vi "IR Polarimeter Software for NIRPol-2.0.vi"() -> ()   [LabVIEW 2017]
uses:
  <vilib>/vision/Image Controls.llb/IMAQ Image.ctl
  <vilib>/Analysis/Matrix/Datatypes/RealMatrix.ctl
  <vilib>/userdefined/High Color/IMAQdx.ctl
  <vilib>/Analysis/baseanly.llb/A x Vector.vi
  <vilib>/Analysis/baseanly.llb/Real A x B.vi
  <vilib>/Instr/_visa.llb/VISA Configure Serial Port (Instr).vi
  <vilib>/Utility/file.llb/Read From Spreadsheet File (DBL).vi
  <vilib>/Utility/file.llb/Write Delimited Spreadsheet (DBL).vi
  <vilib>/gmath/NI_Gmath.lvlib
  <vilib>/Analysis/NI_AALBase.lvlib
  <vilib>/vision/driver/NI_Vision_Acquisition_Software.lvlib
  <vilib>/Analysis/Matrix/NI_Matrix.lvlib
panel:
  out "Abs(cal data - Fit)":dbl[](graph)
  out "Cal Data":dbl[](graph)
  out "Fit":dbl[](graph)
  out "Waveform Chart":dbl(graph)
  out "Numeric":i32
  in  "ROI":i32[](array[numeric])=[155, 255, 103, 203]
  out "IMAQ Session":T1
  out "Camera Handle":T2="cam8"
  in  "Stop Sweeping":bool
  out "Scan Parameters":T3(array[cluster])
  out "cal data and fit":dbl[][][](array[numeric])
  out "Average MM":T4
  out "Dark Img":dbl[][](array[numeric])
  out "Reference Detector Conn":refnum<k21>="RefDetVoltage"
  out "Interface Name":string="img0"
  out "Retarder Motors Driver Output":string
  out "Retarder Motor Driver":refnum<visa-resource-name>
  out "laser VISA Session":refnum<visa-resource-name>
  out "Cal Wavelength":dbl[](array[numeric])
  out "Cal Parameters":dbl[][](array[numeric])
  out "NumWav":dbl=1550.0
  out "Ret Pos":cluster{"Generator":dbl, "Analyzer":dbl}[](array[cluster])
  out "Wavelength List":dbl[](array[numeric])
  out "inverse MM":dbl[][][](array[numeric])
  out "Dark Ref":dbl format="%0.2f"
  out "Reference Detector Reading":string
  out "Reference Detector Value":dbl format="%0.9f"
  out "Image Out":T1
  out "Image Pixels (I16)":i16[][](array[numeric])
  out "Mean":dbl
  out "Minimum":i16
  out "Maximum":i16
  out "Camera Output":i16[][](graph)
  in  "Tab Control":T5(tab)
  in  "Calibrate":bool
  in  "Save calibration file:":path=path "C:/Users/DTS20/Desktop/NIRPOL Revision"
  in  "Load calibration file:":path=path "C:/Users/DTS20/Desktop/NIRPOL Revision/caldata"
  in  "Set Wavelengths:":dbl[][](array[numeric])=[[1550.0]]
  in  "Use User-Defined Retarder Positions?":bool
  in  "Load User-Defined Retarder Positions (optional):":path
  in  "Start Measurement":bool
  in  "Save Mueller Matrix Output To (folder):":path=path "J:/Users/Lisa/foo"
  in  "Use MM Inverse?":bool
  in  "Comments":string
  in  "Use Reference Detector:":bool
  in  "Images to Average":i32=10
  in  "+/-":dbl
  in  "Sweep wavelength?":bool
  in  "Laser On/Off":bool
  in  "Update Camera":bool
  in  "Laser Power [mW]":dbl=6.0 format="%.2f"
  in  "Wavelength [nm]":dbl=1550.0
  in  "Update Laser Source":bool
  in  "PSG Retarder Angle":dbl
  in  "PSA Retarder Angle":dbl
  in  "Update Retarder Angles":bool
  in  "Home Ret Motors":bool
  in  "Exposure [µs]":dbl=1000.0
  in  "Binning":i32=1
  # "Min X"
  # "Max X"
  # "Min Y"
  # "Max Y"
  # "Sweep Wavelength\nDuring Measurement"
  # "AOI"
  # "AOS"
  # "nm"
  # "General Options:"
  # "Laser Control:"
  # "Retarder Motor Control:"
  # "Camera Control"
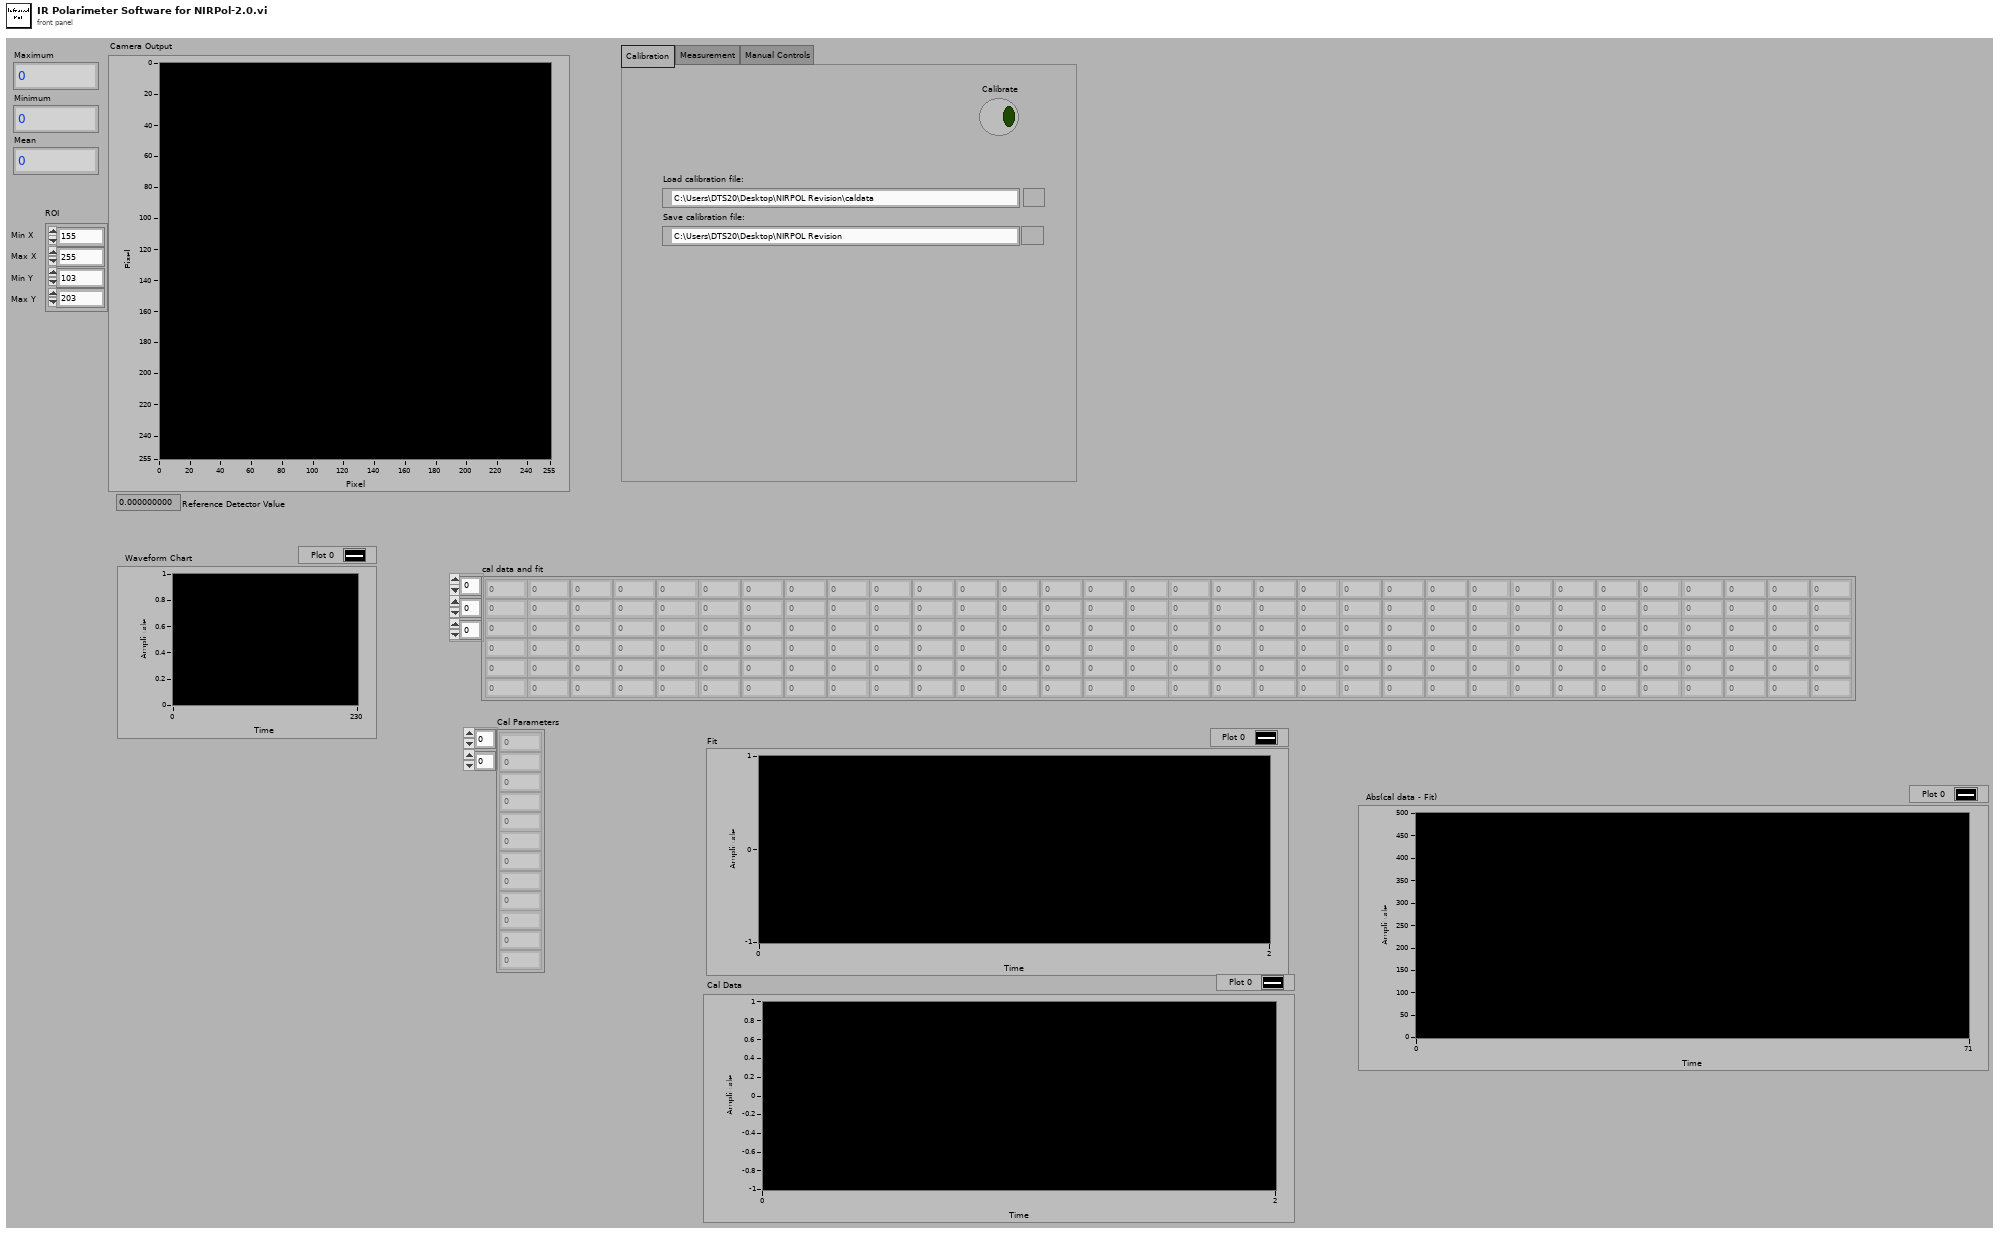
[diagram p1: front panel]
types:
  T1 = typedef "IMAQ Image.ctl" = refnum<image>
  T2 = typedef "IMAQdx.ctl" = refnum<k21>
  T3 = cluster{"Wavelength":dbl, "PSG Angle":dbl, "PSA Angle":dbl}[]
  T4 = typedef "NI_Matrix.lvlib/RealMatrix.ctl" = dbl[][]
  T5 = enum32{"Calibration", "Measurement", "Manual Controls"}
  T6 = enum16{"big-endian, network order", "native, host order", "little-endian"}
  T7 = cluster{"wavelength":dbl, "amplitude":dbl, "gen leakage":dbl, "an leakage":dbl, "generator retardance":dbl, "analyzer retardance":dbl, "gen offset":dbl, "an offset":dbl, "an pol offset":dbl}[]
  T8 = cluster{"Wavelength":dbl, "Camera Arm":dbl, "Source Arm":dbl}[]
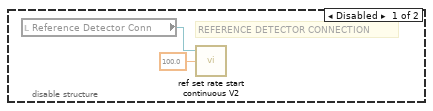
[diagram p2: hidden frame]
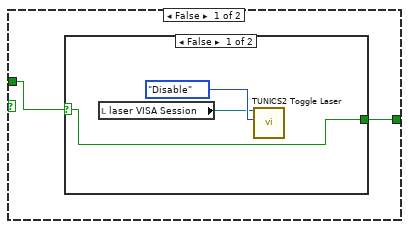
[diagram p3: hidden frame]
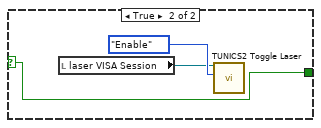
[diagram p4: hidden frame]
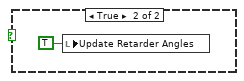
[diagram p5: hidden frame]
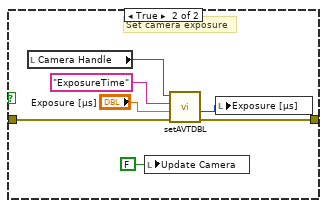
[diagram p6: hidden frame]
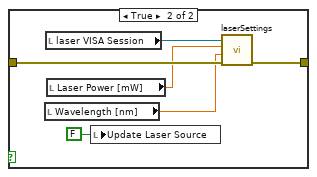
[diagram p7: hidden frame]
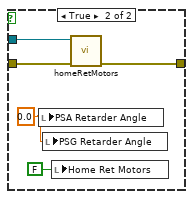
[diagram p9: hidden frame]
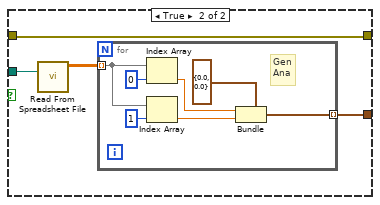
[diagram p10: hidden frame]
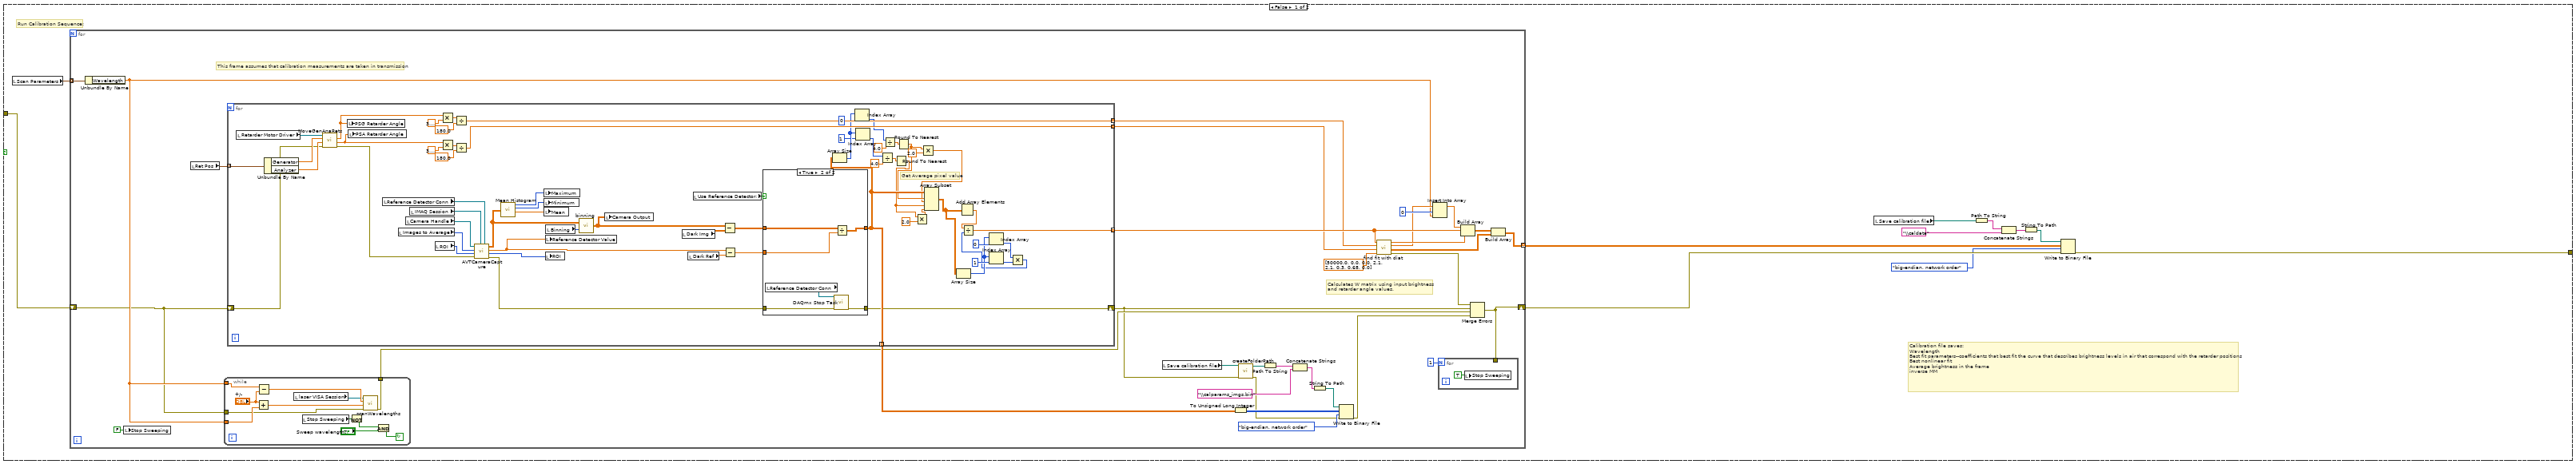
[diagram p11: hidden frame]
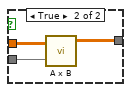
[diagram p13: hidden frame]
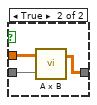
[diagram p14: hidden frame]
diagram:
  # "In This Frame:\n1.) Play a pleasant \"finished\" tone.\n2.) Home retarder motors\n3.) Home arm motors"
  # "In This Frame: Setup for measurement or calibration\n1.) Disable laser to take a dark measurement\n2.) Clear all IMAQ images\n3.) Capture a dark image (to be subtracted from each frame)\n4.) Construct a List of wavelengths and AOI-AOS from user input\n5.) Enable the laser again after a dark measurement\n6.) Load user-defined retarder positions and construct a cluster"
  # "Hidden Constants:"
  # "Display Indicators:"
  # "Numerical Controls:"
  # "Buttons:"
  # "Connections:"
  # "In This Frame:\n1) Initialize the laser\n2) Initialize and home retarder motors\n3) Initialize camera connection\nTODO: Init connection w/ ref detector"
  # "In This Frame:\nContinous Updates are done while the system is setup and prepared for measurement.\n1) Create a bad pixel map\n2) Manually set or home retarder motors\n3) Manually set or home arm motor positions\n4) Manually control laser brightness or wavelength\n5) Continusly Capture camera frames."
  n1 = flat-sequence {
    tunnel: [w38] -> w6
    tunnel: w6 -> [w61]
    tunnel: [w63] -> w2
    tunnel: [w156] -> w5
    tunnel: w2 -> [w146]
    tunnel: w5 -> [w212]
    tunnel: [w211] -> w4
    tunnel: w4 -> [w600]
    frame #0 {
      w16 = 180
      w17 = 3.1416
      w33 = errorcluster {"status"=FALSE, "code"=0, "source"=""} ("error in (no error)")
      w44 = u16 0 items=["None", "XON/XOFF", "RTS/CTS", "XON/XOFF & RTS/CTS", "DTR/DSR", "XON/XOFF & DTR/DSR"] ("flow control (0:none)")
      w47 = u16 10 items=["1.0"=10, "1.5"=15, "2.0"=20] ("stop bits (10: 1 bit)")
      # "RETARDER MOTOR INITIALIZATION"
      # "ILLUMINATION SOURCE CONNECTION"
      # "RETARDER MOTOR CONNECTION"
      # "In This Frame:\nInitialize contact with all hardware needed in system"
      n2 = local read "Camera Handle"() -> (w31:T2)
      n3 = local read "laser VISA Session"() -> (w42:refnum<visa-resource-name>)
      n4 = local read "Retarder Motor Driver"() -> (w43:refnum<visa-resource-name>)
      n5 = call "IMAQ Create"("Image Name"="Grab", "error in (no error)"=w33) -> ("New Image"=→"IMAQ Session":T1, "error out"=w32:errorcluster)  [unwired: 3 in]
      n6 = call <vilib>:"IMAQdx Open Camera.vi"("error in"=w33, "Session In"=w31) -> ("error out"=w36:errorcluster, "Session Out"=w35:T2)  [unwired: 8 in]
      n7 = call "TUNICS2 Toggle Laser.vi"("error in (no error)"=w33, "Laser Output (Disable:0)"=enum16{"Enable", "Disable"}."Enable", "VISA resource name"=w42) -> ("error out"=w39:errorcluster)  [unwired: 3 in, 1 out]
      n8 = call <vilib>:"IMAQdx Configure Grab.vi"("error in"=w36, "Session In"=w35) -> ("error out"=w34:errorcluster)  [unwired: 8 in, 1 out]
      n9 = disable-structure shown="Enabled" {
        frame Disabled {
          # "REFERENCE DETECTOR CONNECTION"
          n10 = local read "Reference Detector Conn"() -> (w57:refnum<k21>)
          n11 = call "ref set rate start continuous V2.vi"("rate (S/s)"=100.0, "task/channels in"=w57) -> ()  [unwired: 1 in, 2 out]
        }
        frame Enabled {
        }
      }
      n12 = local read "Load calibration file:"() -> (w29:path)
      n13 = call-poly "VISA Configure Serial Port"("VISA resource name"=w43, "timeout (10sec)"=u32 1, "termination char\n(0xA = '\\n' = LF)"=u8 10 ("termination char\n(0xA = '\\n' = LF)"), "Enable Termination\nChar (T)"=TRUE ("Enable Termination\nChar (T)"), "baud rate (9600)"=u32 9600, "data bits (8)"=u16 8, "parity (0:none)"=enum16{"None", "Odd", "Even", "Mark", "Space"}."Even", "error in (no error)"=w33, "stop bits (10: 1 bit)"=w47, "flow control (0:none)"=w44) -> ("error out"=w25:errorcluster)  [unwired: 4 in, 1 out]
      n14 = call "LoadCalwDiat.vi"("file (use dialog)"=w29, "error in"=w25) -> ("Calibration params"=w26:T7, "error out"=w28:errorcluster)  [unwired: 2 out]
      n15 = flat-sequence {
        tunnel: w24 -> [w60]
        tunnel: [w58] -> w40
        tunnel: w10 -> [_]
        tunnel: w12 -> [_]
        frame #0 {
          # "01: Gen\n02: Ana"
          # "Homing retarder motors\nSetting arm motors  limits and homing"
          n16 = local read "Retarder Motor Driver"() -> (w59:refnum<visa-resource-name>)
          n17 = call "homeRetMotors.vi"("error in (no error)"=w60, "VISA Refnum in"=w59) -> ("error out"=w58:errorcluster)  [unwired: 9 in]
        }
      }
      n18 = for {
        N: 1 -> [_]
        shift-right: [w52] -> w24
        shift-left: w28 -> [w52]
        tunnel: [w54] -> w23 mode=indexing
        tunnel: [w53] -> w22 mode=indexing
        tunnel: w26 -> [w55] mode=indexing
        n19 = Unbundle By Name(w55) -> ("gen offset"=w54:dbl, "an offset"=w53:dbl)
        n20 = call <vilib>:"Simple Error Handler.vi"("error in (no error)"=w52) -> ()  [unwired: 4 in, 5 out]
      }
      n21 = Negate(x=w23) -> (-x=w21:dbl[])
      n22 = Negate(x=w22) -> (-x=w18:dbl[])
      n23 = Index Array(array=w21, index=0) -> (element=w15:dbl)
      n24 = Index Array(array=w18, index=0) -> (element=w14:dbl)
      n25 = Divide(x=w15, y=w17) -> (x/y=w11:dbl)
      n26 = Divide(x=w14, y=w17) -> (x/y=w13:dbl)
      n27 = Multiply(x=w13, y=w16) -> (x*y=w12:dbl)
      n28 = Multiply(x=w11, y=w16) -> (x*y=w10:dbl)
      n29 = Merge Errors(w39, w33, w40, w34, w32) -> (w38:errorcluster)
      n30 = call <vilib>:"Simple Error Handler.vi"("error in (no error)"=w38) -> ()  [unwired: 4 in, 5 out]
    }
    frame #1 {
      n31 = while {
        shift-right: [w64] -> w63
        shift-left: w61 -> [w87]
        shift-right: [w68] -> _
        shift-left: TRUE ("Laser On/Off") -> [w70]
        i -> [w74]
        stop <- w90 stop-if-true
        # "Camera Capture and Reference Detector Value"
        # "In This Frame:\nUpdate laser power and brightness"
        # "In This Frame:\nUpdate retarder motor angles if maually changed"
        # "In This Frame:\nHome retarder motors"
        n32 = local read "Laser On/Off"() -> (w69:bool)
        n33 = Equal?(x=0, y=w74) -> (x = y?=w72:bool)
        n34 = Equal?(x=w69, y=w70) -> (x = y?=w71:bool)
        n35 = case shown="False" w72 {
          frame False {
          }
          frame True {
            n36 = local write "Update Retarder Angles"(TRUE ("Update Retarder Angles")) -> ()
          }
        }
        n37 = case shown="True" w71 {
          tunnel: w69 -> [w100 w107]
          tunnel: [w99 w107] -> w68
          frame False {
            n38 = case shown="False" w100 {
              selector: w100 -> [w101 w104]
              tunnel: [w101 w104] -> w99
              frame False {
                n39 = local read "laser VISA Session"() -> (w102:refnum<visa-resource-name>)
                n40 = call "TUNICS2 Toggle Laser.vi"("Laser Output (Disable:0)"=enum16{"Enable", "Disable"}."Disable", "VISA resource name"=w102) -> ()  [unwired: 4 in, 2 out]
              }
              frame True {
                n41 = local read "laser VISA Session"() -> (w105:refnum<visa-resource-name>)
                n42 = call "TUNICS2 Toggle Laser.vi"("Laser Output (Disable:0)"=enum16{"Enable", "Disable"}."Enable", "VISA resource name"=w105) -> ()  [unwired: 4 in, 2 out]
              }
            }
          }
          frame True {
          }
        }
        n43 = case shown="False" "Update Camera" {
          tunnel: w87 -> [w109 w116]
          tunnel: [w109 w115] -> w82
          frame False {
          }
          frame True {
            # "Set camera exposure"
            n44 = local read "Camera Handle"() -> (w110:T2)
            n45 = local write "Update Camera"(FALSE ("Update Camera")) -> ()
            n46 = call "setAVTDBL.vi"("error in (no error)"=w116, "Value In"="Exposure [µs]", "ActiveAttribute"="ExposureTime", "Camera Session In"=w110) -> ("error out"=w115:errorcluster, "Value Out"=w112:u32)  [unwired: 5 in, 1 out]
            n47 = local write "Exposure [µs]"(w112) -> ()
          }
        }
        n48 = local read "Retarder Motor Driver"() -> (w93:refnum<visa-resource-name>)
        n49 = local read "Home Ret Motors"() -> (w96:bool)
        n50 = local read "Reference Detector Conn"() -> (w75:refnum<k21>)
        n51 = case shown="False" w96 {
          tunnel: w87 -> [w133 w137]
          tunnel: [w133 w136] -> w94
          tunnel: w93 -> [_ w138]
          frame False {
          }
          frame True {
            w135 = 0.0 ("Analyzer Angle")
            n52 = local write "PSA Retarder Angle"(w135) -> ()
            n53 = local write "PSG Retarder Angle"(w135) -> ()
            n54 = local write "Home Ret Motors"(FALSE ("Home Ret Motors")) -> ()
            n55 = call "homeRetMotors.vi"("error in (no error)"=w137, "VISA Refnum in"=w138) -> ("error out"=w136:errorcluster)  [unwired: 9 in]
          }
        }
        n56 = local read "Images to Average"() -> (w78:i32)
        n57 = local read "Camera Handle"() -> (w77:T2)
        n58 = local read "IMAQ Session"() -> (w76:T1)
        n59 = local read "Binning"() -> (w89:i32)
        n60 = call "AVTCameraCapture.vi"("Reference Detector Conn"=w75, "IMAQ Session"=w76, "error in (no error)"=w82, "ROI In"="ROI", "Images to Average"=w78, "Camera Handle"=w77) -> ("error out"=w65:errorcluster, "ROI Out"=w80:i32[], "Reference Detector Value"=w67:dbl, "Camera Output"=w79:dbl[][])
        "Waveform Chart" <- w67
        n61 = local write "Reference Detector Value"(w67) -> ()
        n62 = local write "ROI"(w80) -> ()
        n63 = call "binning.vi"("Binning"=w89, "Unbinned"=w79) -> ("Binned array"=w88:dbl[][])
        n64 = call "Mean Histogram.vi"("Array"=w79) -> ("max value"=w83:i16, "min value"=w85:i16, "mean val"=w84:dbl)  [unwired: 3 out]
        n65 = case shown="True" "Update Retarder Angles" {
          tunnel: w93 -> [_ w131]
          tunnel: [w124 w130] -> w92
          tunnel: w94 -> [w124 w132]
          frame False {
          }
          frame True {
            n66 = local read "PSG Retarder Angle"() -> (w128:dbl)
            n67 = local read "PSA Retarder Angle"() -> (w127:dbl)
            n68 = local write "Update Retarder Angles"(FALSE ("Update Retarder Angles")) -> ()
            n69 = call "MoveGenAnaRets.vi"("error in (no error)"=w132, "Analyzer In"=w127, "Generator In"=w128, "VISA resource name"=w131) -> ("error out"=w130:errorcluster, "Analyzer Out"=w126:dbl, "Generator Out"=w125:dbl)  [unwired: 1 out]
            n70 = local write "PSA Retarder Angle"(w126) -> ()
            n71 = local write "PSG Retarder Angle"(w125) -> ()
          }
        }
        n72 = local write "Minimum"(w85) -> ()
        n73 = local write "Mean"(w84) -> ()
        n74 = local write "Camera Output"(w88) -> ()
        n75 = local write "Maximum"(w83) -> ()
        n76 = local read "Update Laser Source"() -> (w91:bool)
        n77 = case shown="False" w91 {
          tunnel: w92 -> [w117 w123]
          tunnel: [w117 w122] -> w66
          frame False {
          }
          frame True {
            n78 = local read "Wavelength [nm]"() -> (w120:dbl)
            n79 = local read "laser VISA Session"() -> (w119:refnum<visa-resource-name>)
            n80 = local read "Laser Power [mW]"() -> (w121:dbl)
            n81 = local write "Update Laser Source"(FALSE ("Update Laser Source")) -> ()
            n82 = call "laserSettings.vi"("error in (no error)"=w123, "Wavelength [nm]"=w120, "Laser Power [mW]"=w121, "VISA Refnum in"=w119) -> ("error out"=w122:errorcluster)  [unwired: 1 in, 2 out]
          }
        }
        n83 = local read "Start Measurement"() -> (w98:bool)
        n84 = local read "Calibrate"() -> (w97:bool)
        n85 = Or(x=w98, y=w97) -> (x .or. y?=w90:bool)
        n86 = Merge Errors(w66, w65) -> (w64:errorcluster)
        n87 = call <vilib>:"Simple Error Handler.vi"("error in (no error)"=w64) -> ()  [unwired: 4 in, 5 out]
      }
    }
    frame #2 {
      w144 = 0.0 ("Generator In")
      # "Set scanning parameters:\nThis subVI creates an array of clusters which contain the wavelength and\nscatter angles for each Mueller matrix in the scan"
      # "Capture dark image"
      # "Enable Laser again after the\ndark measurement"
      # "Disable laser to take dark measurement"
      # "If the user desires, they can load an pre-defined retarder angles from an excel doc or csv. Otherwise, a default set of 64 positions is constructed where the PSA rotates 4.9x as fast as the PSG"
      n88 = local read "Retarder Motor Driver"() -> (w143:refnum<visa-resource-name>)
      n89 = call "MoveGenAnaRets.vi"("error in (no error)"=w146, "Analyzer In"=w144, "Generator In"=w144, "VISA resource name"=w143) -> ("error out"=w145:errorcluster, "Analyzer Out"=w148:dbl, "Generator Out"=w147:dbl)  [unwired: 1 out]
      n90 = local write "PSA Retarder Angle"(w148) -> ()
      n91 = local write "PSG Retarder Angle"(w147) -> ()
      n92 = local read "laser VISA Session"() -> (w154:refnum<visa-resource-name>)
      n93 = call "TUNICS2 Toggle Laser.vi"("error in (no error)"=w145, "Laser Output (Disable:0)"=enum16{"Enable", "Disable"}."Disable", "VISA resource name"=w154) -> ("error out"=w151:errorcluster)  [unwired: 3 in, 1 out]
      n94 = flat-sequence {
        tunnel: w151 -> [w167]
        tunnel: [w167] -> w149
        tunnel: w149 -> [w180]
        tunnel: [w179] -> w142
        tunnel: [w185] -> w150
        tunnel: w142 -> [w185]
        frame #0 {
          n95 = Wait (ms)(milliseconds to wait=u32 1000) -> ()  [unwired: 1 out]
        }
        frame #1 {
          # "Save as dark image"
          n96 = local read "Reference Detector Conn"() -> (w174:refnum<k21>)
          n97 = local read "Images to Average"() -> (w177:i32)
          n98 = local read "Camera Handle"() -> (w176:T2)
          n99 = local read "IMAQ Session"() -> (w175:T1)
          n100 = local read "ROI"() -> (w178:i32[])
          n101 = call "AVTCameraCapture.vi"("Reference Detector Conn"=w174, "IMAQ Session"=w175, "error in (no error)"=w180, "ROI In"=w178, "Images to Average"=w177, "Camera Handle"=w176) -> ("error out"=w179:errorcluster, "ROI Out"=w173:i32[], "Reference Detector Value"=w168:dbl, "Camera Output"=w172:dbl[][])
          n102 = local read "Binning"() -> (w181:i32)
          n103 = local write "Dark Ref"(w168) -> ()
          n104 = local write "ROI"(w173) -> ()
          n105 = call "Mean Histogram.vi"("Array"=w172) -> ("max value"=w171:i16, "min value"=w170:i16, "mean val"=w169:dbl)  [unwired: 3 out]
          n106 = local write "Waveform Chart"(w168) -> ()
          n107 = local write "Minimum"(w170) -> ()
          n108 = local write "Maximum"(w171) -> ()
          n109 = local write "Mean"(w169) -> ()
          n110 = call "binning.vi"("Binning"=w181, "Unbinned"=w172) -> ("Binned array"=w182:dbl[][])
          n111 = local write "Camera Output"(w182) -> ()
          n112 = local write "Dark Img"(w182) -> ()
        }
        frame #2 {
          n113 = for {
            N: 10 -> [_]
            tunnel: [w186] -> w183
            i -> [w186]
            n114 = Wait (ms)(milliseconds to wait=u32 1000) -> ()  [unwired: 1 out]
          }
          "Numeric" <- w183
        }
      }
      n115 = call "setScanParams.vi"("error in (no error)"=w150, "Set Wavelengths:"="Set Wavelengths:") -> ("error out"=w141:errorcluster, "Scan Parameters"=→"Scan Parameters":T8)  [unwired: 8 in]
      n116 = flat-sequence {
        tunnel: w141 -> [w163]
        tunnel: [w162] -> w139
        tunnel: [w165] -> w140
        tunnel: w139 -> [w165]
        frame #0 {
          n117 = local read "laser VISA Session"() -> (w160:refnum<visa-resource-name>)
          n118 = call "TUNICS2 Toggle Laser.vi"("error in (no error)"=w163, "Laser Output (Disable:0)"=enum16{"Enable", "Disable"}."Enable", "VISA resource name"=w160) -> ("error out"=w162:errorcluster)  [unwired: 3 in, 1 out]
        }
        frame #1 {
          n119 = Wait (ms)(milliseconds to wait=u32 60000) -> ()  [unwired: 1 out]
        }
      }
      n120 = case shown="False" "Use User-Defined Retarder Positions?" {
        tunnel: [w189 w201] -> w158
        tunnel: "Load User-Defined Retarder Positions (optional):" -> [_ w203]
        tunnel: w140 -> [w188 w200]
        tunnel: [w188 w200] -> w156
        frame False {
          n121 = for {
            N: 64 -> [w198]
            tunnel: [w191] -> w189 mode=indexing
            i -> [w196]
            n122 = Divide(x=360.0, y=w198) -> (x/y=w197:dbl)
            n123 = Multiply(x=w197, y=w196) -> (x*y=w194:dbl)
            n124 = Multiply(x=w194, y=4.9) -> (x*y=w193:dbl)
            n125 = Bundle(cluster=cluster{"x":dbl, "x 2":dbl} {"x"=0.0, "x 2"=0.0} ("input cluster"), "x"=w193, "x 2"=w194) -> (w191:cluster{"x":dbl, "x 2":dbl})
          }
        }
        frame True {
          n126 = call-poly <vilib>:"Read From Spreadsheet File.vi"("file path (dialog if empty)"=w203) -> ("all rows"=w202:dbl[][])  [unwired: 6 in, 4 out]
          n127 = for {
            tunnel: w202 -> [w208] mode=indexing
            tunnel: [w204] -> w201 mode=indexing
            # "Gen\nAna"
            n128 = Index Array(array=w208, index=0) -> (element=w206:dbl)
            n129 = Index Array(array=w208, index=1) -> (element=w205:dbl)
            n130 = Bundle(cluster=cluster{"x":dbl, "x 2":dbl} {"x"=0.0, "x 2"=0.0} ("input cluster"), "x"=w206, "x 2"=w205) -> (w204:cluster{"x":dbl, "x 2":dbl})
          }
        }
      }
      n131 = local write "Ret Pos"(w158) -> ()
    }
    frame #3 {
      # "In This Frame: Run a measurement or a calibration"
      n132 = local read "Start Measurement"() -> (w213:bool)
      n133 = case shown="True" w213 {
        tunnel: w212 -> [w224 w365]
        tunnel: [w220 w359] -> w211
        frame False {
          # "Calibration file saves:\nWavelength\nBest fit parameters--coefficients that best fit the curve that describes brightness levels in air that correspond with the retarder positions\nBest nonlinear fit\nAverage brightness in the frame\ninverse MM"
          # "Run Calibration Sequence:"
          n134 = local read "Scan Parameters"() -> (w219:T3)
          n135 = for {
            tunnel: [w249] -> w221 mode=indexing
            shift-right: [w240] -> w223
            shift-left: w224 -> [w227]
            tunnel: w219 -> [w244] mode=indexing
            # "Calculates W matrix using input brightness\nand retarder angle values."
            # "This frame assumes that calibration measurements are taken in transmission"
            n136 = Unbundle By Name(w244) -> ("Wavelength"=w242:dbl)
            n137 = local write "Stop Sweeping"(FALSE ("stop scanning")) -> ()
            n138 = local read "Ret Pos"() -> (w254:cluster{"Generator":dbl, "Analyzer":dbl}[])
            n139 = while {
              tunnel: w242 -> [w269]
              tunnel: w242 -> [w267]
              tunnel: w227 -> [w259]
              tunnel: [w258] -> w226
              stop <- w261 continue-if-true
              n140 = Add(x="+/-", y=w269) -> (x+y=w268:dbl)
              n141 = Subtract(x=w267, y="+/-") -> (x-y=w265:dbl)
              n142 = local read "laser VISA Session"() -> (w260:refnum<visa-resource-name>)
              n143 = local read "Stop Sweeping"() -> (w264:bool)
              n144 = Not(x=w264) -> (.not. x?=w263:bool)
              n145 = call "scanWavelengths.vi"("error in (no error)"=w259, "Start Wavelength [nm]"=w268, "End Wavelength [nm]"=w265, "VISA Refnum in"=w260) -> ("error out"=w258:errorcluster)  [unwired: 7 in]
              n146 = And(x=w263, y="Sweep wavelength?") -> (x .and. y?=w261:bool)
            }
            n147 = for {
              tunnel: [w330] -> w252 mode=indexing
              shift-right: [w271] -> w225
              shift-left: w227 -> [w302]
              tunnel: w254 -> [w318] mode=indexing
              tunnel: [w312] -> w245 mode=indexing
              tunnel: [w308] -> w246 mode=indexing
              tunnel: [w284] -> w238 mode=indexing
              # "Get Average pixel value"
              n148 = local read "Retarder Motor Driver"() -> (w305:refnum<visa-resource-name>)
              n149 = Unbundle By Name(w318) -> ("Generator"=w304:dbl, "Analyzer"=w303:dbl)
              n150 = call "MoveGenAnaRets.vi"("error in (no error)"=w302, "Analyzer In"=w303, "Generator In"=w304, "VISA resource name"=w305) -> ("error out"=w291:errorcluster, "Analyzer Out"=w300:dbl, "Generator Out"=w301:dbl)  [unwired: 1 out]
              n151 = local write "PSG Retarder Angle"(w301) -> ()
              n152 = local write "PSA Retarder Angle"(w300) -> ()
              n153 = local read "Reference Detector Conn"() -> (w270:refnum<k21>)
              n154 = local read "Images to Average"() -> (w293:i32)
              n155 = local read "Camera Handle"() -> (w294:T2)
              n156 = local read "IMAQ Session"() -> (w295:T1)
              n157 = local read "ROI"() -> (w292:i32[])
              n158 = Multiply(x=w301, y=3.141592653589793) -> (x*y=w314:dbl)
              n159 = Multiply(x=w300, y=3.141592653589793) -> (x*y=w310:dbl)
              n160 = Divide(x=w314, y=180.0) -> (x/y=w312:dbl)
              n161 = Divide(x=w310, y=180.0) -> (x/y=w308:dbl)
              n162 = call "AVTCameraCapture.vi"("Reference Detector Conn"=w270, "IMAQ Session"=w295, "error in (no error)"=w291, "ROI In"=w292, "Images to Average"=w293, "Camera Handle"=w294) -> ("error out"=w289:errorcluster, "ROI Out"=w297:i32[], "Reference Detector Value"=w290:dbl, "Camera Output"=w299:dbl[][])
              n163 = call "Mean Histogram.vi"("Array"=w299) -> ("max value"=w316:i16, "min value"=w317:i16, "mean val"=w296:dbl)  [unwired: 3 out]
              n164 = local write "Maximum"(w316) -> ()
              n165 = local write "Minimum"(w317) -> ()
              n166 = local write "Mean"(w296) -> ()
              n167 = local write "Reference Detector Value"(w290) -> ()
              n168 = local write "ROI"(w297) -> ()
              n169 = local read "Binning"() -> (w306:i32)
              n170 = call "binning.vi"("Binning"=w306, "Unbinned"=w299) -> ("Binned array"=w298:dbl[][])
              n171 = local write "Camera Output"(w298) -> ()
              n172 = local read "Dark Img"() -> (w307:dbl[][])
              n173 = local read "Dark Ref"() -> (w322:dbl)
              n174 = local read "Use Reference Detector:"() -> (w319:bool)
              n175 = Subtract(x=w298, y=w307) -> (x-y=w323:dbl[][])
              n176 = Subtract(x=w290, y=w322) -> (x-y=w321:dbl)
              n177 = case shown="True" w319 {
                tunnel: w323 -> [w332 w338]
                tunnel: w321 -> [_ w337]
                tunnel: [w332 w336] -> w284
                tunnel: w289 -> [w331 w335]
                tunnel: [w331 w333] -> w271
                frame False {
                }
                frame True {
                  n178 = local read "Reference Detector Conn"() -> (w334:refnum<k21>)
                  n179 = call <vilib>:"DAQmx Stop Task.vi"("task/channels in"=w334, "error in"=w335) -> ("error out"=w333:errorcluster)  [unwired: 12 in, 1 out]
                  n180 = Divide(x=w338, y=w337) -> (x/y=w336:dbl[][])
                }
              }
              n181 = Array Size(array=w284) -> (size(s)=w288:i32[])
              n182 = Index Array(array=w288, index=0) -> (element=w282:i32)
              n183 = Index Array(array=w288, index=1) -> (element=w280:i32)
              n184 = Divide(x=w280, y=4.0) -> (x/y=w279:dbl)
              n185 = Divide(x=w282, y=4.0) -> (x/y=w278:dbl)
              n186 = Round To Nearest(number=w279) -> (nearest integer value=w273:dbl)
              n187 = Round To Nearest(number=w278) -> (nearest integer value=w277:dbl)
              n188 = Multiply(x=w273, y=2.0) -> (x*y=w272:dbl)
              n189 = Multiply(x=w277, y=2.0) -> (x*y=w275:dbl)
              n190 = Array Subset "Array Subset"(array=w284, index (row)=w277, length (row)=w275, index (col)=w273, length (col)=w272) -> (w285:dbl[][])
              n191 = Array Size(array=w285) -> (size(s)=w327:i32[])
              n192 = Add Array Elements(numeric array=w285) -> (sum=w320:dbl)
              n193 = Index Array(array=w327, index=0) -> (element=w325:i32)
              n194 = Index Array(array=w327, index=1) -> (element=w326:i32)
              n195 = Multiply(x=w325, y=w326) -> (x*y=w324:i32)
              n196 = Divide(x=w320, y=w324) -> (x/y=w330:dbl)
            }
            n197 = local read "Save calibration file:"() -> (w236:path)
            n198 = To Unsigned Long Integer(number=w238) -> (unsigned 32bit integer=w237:u32[][][])
            n199 = call "createFolderPath.vi"("error in (no error)"=w225, "File Path Control"=w236) -> ("error out"=w229:errorcluster, "Path"=w235:path)  [unwired: 8 in]
            n200 = Path To String(path=w235) -> (string=w234:string)
            n201 = Concatenate Strings(w234, "\\calparams_imgs.bin") -> (w232:string)
            n202 = String To Path(string=w232) -> (path=w231:path)
            n203 = Write to Binary File(file (use dialog)=w231, data=w237, error in=w229, 9:T6."big-endian, network order" ("byte order (0:big-endian, network order)")) -> (error out=w228:errorcluster)  [unwired: 2 in, 2 out]
            n204 = call "find fit with diat.vi"("initial parameters"=dbl[] [50000.0, 0.0, 0.0, 2.1, 2.1, 0.3, 0.68, 0.0], "t2"=w246, "t1"=w245, "Y"=w252) -> ("error out"=w239:errorcluster, "inverse MM"=w248:dbl[][], "best fit parameters"=w250:dbl[], "best nonlinear fit"=w251:dbl[])
            n205 = Insert Into Array(array=w250, index=0, new element=w242) -> (w256:dbl[])
            n206 = Build Array(w256, w252, w251) -> (w247:dbl[][])
            n207 = Merge Errors(w239, w225, w226, w228) -> (w240:errorcluster)
            n208 = for {
              N: 1 -> [_]
              tunnel: w240 -> [_]
              n209 = local write "Stop Sweeping"(TRUE ("stop scanning")) -> ()
            }
            n210 = Build Array(w247, w248) -> (w249:dbl[][][])
          }
          n211 = local read "Save calibration file:"() -> (w218:path)
          n212 = Path To String(path=w218) -> (string=w217:string)
          n213 = Concatenate Strings(w217, "\\caldata") -> (w215:string)
          n214 = String To Path(string=w215) -> (path=w214:path)
          n215 = Write to Binary File(file (use dialog)=w214, data=w221, error in=w223, 9:T6."big-endian, network order" ("byte order (0:big-endian, network order)")) -> (error out=w220:errorcluster)  [unwired: 2 in, 2 out]
        }
        frame True {
          # "Load calibration data and save to calibration paramenters:"
          # "Note: not currently set up to push out the correct system setup data"
          # "TODO: Correct Reference Detector data type: needs to be a 1D array, is a double"
          # "Run Measurement Sequence:"
          n216 = local read "Load calibration file:"() -> (w366:path)
          n217 = call "LoadCalwDiat.vi"("file (use dialog)"=w366, "error in"=w365) -> ("Calibration params"=w348:T7, "cal data and fit"=w347:dbl[][][], "inverse MM"=w364:dbl[][][], "error out"=w350:errorcluster)
          "cal data and fit" <- w347
          n218 = for {
            N: 1 -> [_]
            shift-right: [w369] -> w362
            shift-left: w350 -> [w369]
            tunnel: [w375] -> w358 mode=indexing
            tunnel: [w374] -> w357 mode=indexing
            tunnel: [w373] -> w356 mode=indexing
            tunnel: [w368] -> w355 mode=indexing
            tunnel: [w367] -> w354 mode=indexing
            tunnel: [w372] -> w353 mode=indexing
            tunnel: [w371] -> w352 mode=indexing
            tunnel: [w370] -> w351 mode=indexing
            tunnel: [w376] -> w360 mode=indexing
            tunnel: w348 -> [w377] mode=indexing
            n219 = Unbundle By Name(w377) -> ("wavelength"=w376:dbl, "amplitude"=w375:dbl, "gen leakage"=w374:dbl, "an leakage"=w373:dbl, "generator retardance"=w368:dbl, "analyzer retardance"=w367:dbl, "gen offset"=w372:dbl, "an offset"=w371:dbl, "an pol offset"=w370:dbl)
            n220 = call <vilib>:"Simple Error Handler.vi"("error in (no error)"=w369) -> ()  [unwired: 4 in, 5 out]
          }
          "Cal Wavelength" <- w360
          n221 = Build Array(w358, w357, w356, w355, w354, w353, w352, w351) -> (→"Cal Parameters":dbl[][])
          n222 = Index Array(array=w347, index (dim 0)=0 ("index (page)"), index (dim 1)=0 ("index (row)")) -> (element=w342:dbl[])  [unwired: 1 in]
          "Cal Data" <- w342
          n223 = Index Array(array=w347, index (dim 0)=0 ("index (page)"), index (dim 1)=1 ("disabled index (row)")) -> (element=w341:dbl[])  [unwired: 1 in]
          "Fit" <- w341
          n224 = local write "inverse MM"(w364) -> ()
          n225 = Subtract(x=w342, y=w341) -> (x-y=w340:dbl[])
          n226 = Absolute Value(x=w340) -> (abs(x)=→"Abs(cal data - Fit)":dbl[])
          n227 = local read "Scan Parameters"() -> (w363:T3)
          n228 = for {
            tunnel: w363 -> [w398] mode=indexing
            tunnel: w362 -> [w399]
            tunnel: [w402] -> w359
            w430 = 0 ("index")
            w463 = i16 2 ("precision (6)")
            # "Set laser to the correct wavelength"
            # "Compares input wavelength to calibrated \nwavelengths to fit values for calibraton \nparameters if the input isn't an exact vlaue \nthat has been measured before."
            # "W Inv Matrix"
            # "Output Files"
            # "Inverse Mueller Matrix Calculations"
            # "Applies Calibration Parameters"
            # "Calculates Average Mueller Matrix"
            # "imgs = binary copy of live image seen on front panel\nmm = bin file of MM\nref = reference detector reading corresponding to imgs, uncorrected by darkRef\ndarkRef = dark reference detector reading\ndarkImg = dark image corresponding to reading"
            # "Camera Capture Sequence:\nImage averaging and binning\nNOTE: binning not an available feature in the FLIR Pheonix camera"
            n229 = local read "laser VISA Session"() -> (w391:refnum<visa-resource-name>)
            n230 = Unbundle By Name(w398) -> ("Wavelength"=w385:dbl)  [unwired: 2 out]
            n231 = local write "Stop Sweeping"(FALSE ("stop scanning")) -> ()
            n232 = call <instrlib>:"TUNICS2 Set Wavelength.vi"("error in (no error)"=w399, "Wavelength [nm]"=w385, "VISA resource name"=w391) -> ("error out"=w378:errorcluster)  [unwired: 3 in, 1 out]
            n233 = while {
              tunnel: w385 -> [w474]
              tunnel: w385 -> [w472]
              tunnel: w391 -> [w465]
              stop <- w468 continue-if-true
              n234 = local read "+/-"() -> (w471:dbl)
              n235 = Subtract(x=w474, y=w471) -> (x-y=w473:dbl)
              n236 = Add(x=w471, y=w472) -> (x+y=w470:dbl)
              n237 = call "scanWavelengths.vi"("Start Wavelength [nm]"=w470, "End Wavelength [nm]"=w473, "VISA Refnum in"=w465) -> ()  [unwired: 8 in, 1 out]
              n238 = local read "Sweep wavelength?"() -> (w469:bool)
              n239 = local read "Stop Sweeping"() -> (w467:bool)
              n240 = Not(x=w467) -> (.not. x?=w466:bool)
              n241 = And(x=w466, y=w469) -> (x .and. y?=w468:bool)
            }
            n242 = local read "Ret Pos"() -> (w449:cluster{"Generator":dbl, "Analyzer":dbl}[])
            n243 = for {
              tunnel: [w527] -> w390 mode=indexing
              tunnel: [w536] -> w386 mode=indexing
              tunnel: [w535] -> w392 mode=indexing
              shift-right: [w538] -> w412
              shift-left: w378 -> [w539]
              tunnel: w449 -> [w537] mode=indexing
              tunnel: [w529] -> w439 mode=indexing
              tunnel: [w530] -> w438 mode=indexing
              # "This FOR loop moves arms to proper positions & adjusts wavelength"
              n244 = flat-sequence {
                tunnel: w539 -> [w541]
                tunnel: w537 -> [w547]
                tunnel: [w540] -> w534
                tunnel: [w542] -> w533
                tunnel: [w543] -> w531
                tunnel: w534 -> [w552]
                tunnel: w533 -> [w557]
                tunnel: [w550] -> w532
                tunnel: w531 -> [w559]
                tunnel: [w558] -> w530
                tunnel: [w556] -> w529
                tunnel: [w551] -> w528
                tunnel: [w589] -> w538
                tunnel: [w584] -> w527
                tunnel: [w587] -> w536
                tunnel: [w581] -> w535
                tunnel: w532 -> [w581]
                tunnel: w528 -> [w589]
                frame #0 {
                  n245 = Unbundle By Name(w547) -> ("Generator"=w545:dbl, "Analyzer"=w544:dbl)
                  n246 = local read "Retarder Motor Driver"() -> (w546:refnum<visa-resource-name>)
                  n247 = call "MoveGenAnaRets.vi"("error in (no error)"=w541, "Analyzer In"=w544, "Generator In"=w545, "VISA resource name"=w546) -> ("error out"=w540:errorcluster, "Analyzer Out"=w542:dbl, "Generator Out"=w543:dbl)  [unwired: 1 out]
                  n248 = local write "PSG Retarder Angle"(w543) -> ()
                  n249 = local write "PSA Retarder Angle"(w542) -> ()
                }
                frame #1 {
                  n250 = expression code="(x/180.0)*pi" "degrees to radians"(w557) -> (w556:dbl)
                  n251 = expression code="(x/180.0)*pi" "degrees to radians"(w559) -> (w558:dbl)
                  n252 = local read "Images to Average"() -> (w553:i32)
                  n253 = local read "ROI"() -> (w549:i32[])
                  n254 = call "setAVTROI.vi"("Acquisition Window"=w549) -> ("initialized array"=w548:u32[][])  [unwired: 7 in, 3 out]
                  n255 = for {
                    N: w553 -> [_]
                    shift-right: [w562] -> w551
                    shift-left: w552 -> [w565]
                    shift-right: [w577] -> w554
                    shift-left: w548 -> [w576]
                    tunnel: w553 -> [w575]
                    n256 = local read "Camera Handle"() -> (w571:T2)
                    n257 = local read "Reference Detector Conn"() -> (w561:refnum<k21>)
                    n258 = local read "IMAQ Session"() -> (w570:T1)
                    n259 = call <vilib>:"IMAQdx Grab.vi"("error in"=w565, "Image In"=w570, "Session In"=w571) -> ("error out"=w573:errorcluster, "Image Out"=w572:T1)  [unwired: 5 in, 2 out]
                    n260 = call "getRefData.vi"("error in (no error)"=w565, "Task In"=w561) -> ("error out"=w564:errorcluster, "mean"=w560:dbl)  [unwired: 2 in, 2 out]
                    n261 = local write "Image Out"(w572) -> ()
                    n262 = call "IMAQ ImageToArray"("error in (no error)"=w573, "Image"=w572) -> ("error out"=w569:errorcluster, "Image Pixels (I16)"=w567:i16[][])  [unwired: 2 in, 3 out]
                    n263 = local write "Waveform Chart"(w560) -> ()
                    n264 = local write "Reference Detector Value"(w560) -> ()
                    n265 = local read "ROI"() -> (w568:i32[])
                    n266 = call "setAVTROI.vi"("error in (no error)"=w569, "Acquisition Window"=w568, "Array"=w567) -> ("error out"=w563:errorcluster, "ROI"=w566:i16[][])  [unwired: 5 in, 2 out]
                    n267 = Divide(x=w566, y=w575) -> (x/y=w574:dbl[][])
                    n268 = call "Mean Histogram.vi"("Array"=w566) -> ("max value"=w578:i16, "min value"=w580:i16, "mean val"=w579:dbl)  [unwired: 3 out]
                    n269 = Merge Errors(w564, w563) -> (w562:errorcluster)
                    n270 = local write "Mean"(w579) -> ()
                    n271 = Add(x=w574, y=w576) -> (x+y=w577:dbl[][])
                    n272 = local write "Maximum"(w578) -> ()
                    n273 = local write "Minimum"(w580) -> ()
                  }
                  n274 = local read "Binning"() -> (w555:i32)
                  n275 = call "binning.vi"("Binning"=w555, "Unbinned"=w554) -> ("Binned array"=w550:dbl[][])
                  n276 = local write "Camera Output"(w550) -> ()
                }
                frame #2 {
                  n277 = local read "Dark Img"() -> (w582:dbl[][])
                  n278 = local read "Reference Detector Value"() -> (w587:dbl)
                  n279 = Subtract(x=w581, y=w582) -> (x-y=w583:dbl[][])
                  n280 = local read "Use Reference Detector:"() -> (w586:bool)
                  n281 = local read "Dark Ref"() -> (w588:dbl)
                  n282 = Subtract(x=w587, y=w588) -> (x-y=w585:dbl)
                  n283 = case shown="True" w586 {
                    tunnel: w583 -> [w590 w593]
                    tunnel: w585 -> [_ w592]
                    tunnel: [w590 w591] -> w584
                    frame False {
                    }
                    frame True {
                      n284 = Divide(x=w593, y=w592) -> (x/y=w591:dbl[][])
                    }
                  }
                }
              }
            }
            n285 = Build Array(w385) -> (w433:dbl[])
            n286 = local read "Cal Wavelength"() -> (w434:dbl[])
            n287 = local read "Cal Parameters"() -> (w442:dbl[][])
            n288 = for {
              tunnel: [w525] -> w441 mode=indexing
              tunnel: w433 -> [_]
              tunnel: w442 -> [w524] mode=indexing
              tunnel: w434 -> [w523]
              n289 = call <vilib>:"Interpolate 1D.vi"("X"=w523, "Y"=w524) -> ("yi"=w526:dbl[])  [unwired: 7 in, 2 out]
              n290 = Index Array(array=w526) -> (element=w525:dbl)  [unwired: 1 in]
            }
            n291 = Interleave 1D Arrays(w438, w439) -> (w440:dbl[])
            n292 = call "get w matrix with diat.vi"("X"=w440, "a"=w441) -> ("w inverse matrix"=w384:dbl[][])
            n293 = Array Size(array=w390) -> (size(s)=w445:i32[])
            n294 = for {
              N: 4 -> [w479]
              tunnel: [w478] -> w429 mode=indexing
              tunnel: w434 -> [w477]
              tunnel: w433 -> [w476]
              i -> [w480]
              # "input wavelength interpoation to cal file"
              n295 = for {
                N: w479 -> [_]
                tunnel: w480 -> [w485]
                tunnel: [w482] -> w478 mode=indexing
                tunnel: w477 -> [w481]
                tunnel: w476 -> [_]
                i -> [w486]
                n296 = local read "inverse MM"() -> (w487:dbl[][][])
                n297 = Index Array(array=w487, index (dim 1)=w485, index (dim 2)=w486) -> (element=w484:dbl[])  [unwired: 1 in]
                n298 = call <vilib>:"Interpolate 1D.vi"("X"=w481, "Y"=w484) -> ("yi"=w483:dbl[])  [unwired: 7 in, 2 out]
                n299 = for {
                  tunnel: w483 -> [w488] mode=indexing
                  tunnel: [w488] -> w482
                }
              }
            }
            n300 = Index Array(array=w445, index=1) -> (element=w446:i32)
            n301 = Index Array(array=w445, index=2) -> (element=w444:i32)
            n302 = for {
              N: w446 -> [_]
              tunnel: w444 -> [w500]
              tunnel: w390 -> [w499]
              tunnel: [w498] -> w427 mode=indexing
              tunnel: "Use MM Inverse?" -> [w497]
              shift-right: [w495] -> w431
              shift-left: dbl[][] [[0.0, 0.0, 0.0, 0.0], [0.0, 0.0, 0.0, 0.0], [0.0, 0.0, 0.0, 0.0], [0.0, 0.0, 0.0, 0.0]] -> [w496]
              tunnel: w384 -> [w494]
              tunnel: w429 -> [w493]
              i -> [w501]
              n303 = for {
                N: w500 -> [_]
                tunnel: w501 -> [w507]
                tunnel: w499 -> [w513]
                tunnel: [w512] -> w498 mode=indexing
                tunnel: w497 -> [w511]
                shift-right: [w508] -> w495
                shift-left: w496 -> [w509]
                tunnel: w494 -> [w503]
                tunnel: w493 -> [w502]
                i -> [w506]
                # "W Inv Matrix"
                n304 = Index Array(array=w513, index (dim 1)=w507, index (dim 2)=w506) -> (element=w505:dbl[])  [unwired: 1 in]
                n305 = call-poly <vilib>:"A x B.vi"("Vector"=w505, "A"=w503) -> ("A x Vector"=w504:dbl[])  [unwired: 1 out]
                n306 = Decimate 1D Array(w504) -> (w518:dbl[], w517:dbl[], w515:dbl[], w516:dbl[])
                n307 = Build Array(w518, w517, w515, w516) -> (w514:dbl[][])
                n308 = Transpose 2D Array(2D array=w514) -> (transposed array=w510:dbl[][])
                n309 = case shown="False" w511 {
                  tunnel: [w519 w522] -> w512
                  tunnel: w510 -> [w519 w521]
                  tunnel: w502 -> [_ w520]
                  frame False {
                  }
                  frame True {
                    n310 = call-poly <vilib>:"A x B.vi"("B"=w521, "A"=w520) -> ("A x B"=w522:T4)  [unwired: 1 out]
                  }
                }
                n311 = Add(x=w510, y=w509) -> (x+y=w508:dbl[][])
              }
            }
            n312 = Divide(x=w392, y=1 ("index")) -> (x/y=w424:dbl[][][])
            n313 = To Long Integer(number=w424) -> (32bit integer=w421:i32[][][])
            n314 = Unbundle By Name(w398) -> ("Wavelength"=w397:dbl, "PSG Angle"=w396:dbl, "PSA Angle"=w395:dbl)
            n315 = Index Array(array=w431, index (row)=w430, index (col)=w430) -> (element=w432:dbl)
            n316 = Divide(x=w431, y=w432) -> (x/y=w437:dbl[][])
            n317 = case shown="False" "Use MM Inverse?" {
              tunnel: w437 -> [w489 w492]
              tunnel: w429 -> [_ w491]
              tunnel: [w489 w490] -> w428
              frame False {
              }
              frame True {
                n318 = call-poly <vilib>:"A x B.vi"("B"=w492, "A"=w491) -> ("A x B"=w490:T4)  [unwired: 1 out]
              }
            }
            "Average MM" <- w428
            n319 = Insert Into Array(array=w386, index=0, new element=w385) -> (w383:dbl[])
            n320 = call "createFolderPath.vi"("File Path Control"="Save Mueller Matrix Output To (folder):") -> ("Path"=w400:path)  [unwired: 9 in, 1 out]
            n321 = Number To Fractional String(number=w397, precision (6)=w463) -> (F-format string=w460:string)  [unwired: 2 in]
            n322 = Number To Fractional String(number=w396, precision (6)=w463) -> (F-format string=w458:string)  [unwired: 2 in]
            n323 = Number To Fractional String(number=w395, precision (6)=w463) -> (F-format string=w459:string)  [unwired: 2 in]
            n324 = Path To String(path=w400) -> (string=w380:string)
            n325 = Concatenate Strings(w380, "\\PSG" ("string"), w458, "PSA" ("string"), w459, "wav" ("string"), w460) -> (w406:string)
            n326 = local read "Dark Img"() -> (w423:dbl[][])
            n327 = local read "Dark Ref"() -> (w422:dbl)
            n328 = Divide(x=w427, y=65000 ("index")) -> (x/y=w411:dbl[][][][])
            n329 = To Long Integer(number=w423) -> (32bit integer=w415:i32[][])
            n330 = To Long Integer(number=w422) -> (32bit integer=w416:i32)
            n331 = Concatenate Strings(w406, "imgs.bin" ("string")) -> (w454:string)
            n332 = Concatenate Strings(w406, "darkRef.bin" ("string")) -> (w450:string)
            n333 = Concatenate Strings(w406, "mm.bin" ("string")) -> (w462:string)
            n334 = Concatenate Strings(w406, "info.txt" ("string")) -> (w408:string)
            n335 = Concatenate Strings(w406, "darkImg.bin" ("string")) -> (w453:string)
            n336 = Concatenate Strings(w380, "\\ref_readings.dat" ("string")) -> (w381:string)
            n337 = String To Path(string=w454) -> (path=w419:path)
            n338 = String To Path(string=w450) -> (path=w417:path)
            n339 = String To Path(string=w381) -> (path=w389:path)
            n340 = String To Path(string=w462) -> (path=w409:path)
            n341 = String To Path(string=w408) -> (path=w407:path)
            n342 = String To Path(string=w453) -> (path=w414:path)
            n343 = call-poly <vilib>:"Write Delimited Spreadsheet.vi"("file path (dialog if empty)"=w389, "1D data"=w383, "transpose? (no:F)"=TRUE) -> ("error out"=w388:errorcluster)  [unwired: 11 in, 1 out]
            n344 = Write to Binary File(file (use dialog)=w419, data=w421) -> (error out=w420:errorcluster)  [unwired: 4 in, 2 out]
            n345 = Write to Binary File(file (use dialog)=w417, data=w416) -> (error out=w418:errorcluster)  [unwired: 4 in, 2 out]
            n346 = Write to Binary File(file (use dialog)=w414, data=w415) -> (error out=w413:errorcluster)  [unwired: 4 in, 2 out]
            n347 = Write to Binary File(file (use dialog)=w409, data=w411, error in=w412) -> (error out=w410:errorcluster)  [unwired: 3 in, 2 out]
            n348 = Write to Text File(file (use dialog)=w407, text="Comments") -> (error out=w403:errorcluster)  [unwired: 2 in, 2 out]
            n349 = Merge Errors "Merge Errors"(w413, w418, w420, w388, w410, w403) -> (w402:errorcluster)
            n350 = for {
              N: 1 -> [_]
              n351 = local write "Stop Sweeping"(TRUE ("stop scanning")) -> ()
            }
          }
        }
      }
    }
    frame #4 {
      w599 = 0.0 ("Generator Angle")
      w602 = FALSE ("Run Scan")
      # "End Camera and IMAQ Session"
      # "Home retarder and arm motors:"
      # "Un-Press measurement buttons:"
      # "Play a tone indicating measurement is complete."
      n352 = local read "Retarder Motor Driver"() -> (w601:refnum<visa-resource-name>)
      n353 = local write "PSA Retarder Angle"(w599) -> ()
      n354 = local write "PSG Retarder Angle"(w599) -> ()
      n355 = local write "Start Measurement"(w602) -> ()
      n356 = local write "Calibrate"(w602) -> ()
      n357 = call "homeRetMotors.vi"("error in (no error)"=w600, "VISA Refnum in"=w601) -> ("error out"=w594:errorcluster)  [unwired: 9 in]
      n358 = call <vilib>:"Beep.vi"("use system alert? (T)"=TRUE, "duration (msec)"=u32 500, "frequency (Hz)"=u32 2200) -> ()  [unwired: 9 in]
      n359 = local read "Camera Handle"() -> (w598:T2)
      n360 = call <vilib>:"IMAQdx Close Camera.vi"("error in"=w594, "Session In"=w598) -> ("error out"=w597:errorcluster)  [unwired: 9 in]
      n361 = local read "IMAQ Session"() -> (w596:T1)
      n362 = call "IMAQ Dispose"("Image"=w596, "error in (no error)"=w597) -> ("error out"=w595:errorcluster)  [unwired: 4 in]
      n363 = call <vilib>:"Simple Error Handler.vi"("error in (no error)"=w595) -> ()  [unwired: 4 in, 5 out]
    }
  }
  "laser VISA Session" <- refnum<visa-resource-name> "GPIB1::10::INSTR" ("laser VISA Session")
  "Retarder Motor Driver" <- refnum<visa-resource-name> "COM6" ("VISA resource name")
  "Interface Name" <- "img0" ("Interface Name")
  "Reference Detector Conn" <- refnum<k21> "MyVoltageTask" ("DAQmx Task Name")
  "Camera Handle" <- T2 "cam10" ("Session In")
